vi "Just video.vi"() -> ()   [LabVIEW 2014]
uses:
  <vilib>/Platform/TimedLoop/XDataNode/wakeup.ctl
  <vilib>/Platform/TimedLoop/XDataNode/XDNodeRunTimeDep.lvlib
  <vilib>/Platform/TimedLoop/XDataNode/nitl_modes.ctl
  <vilib>/Platform/TimedLoop/XDataNode/timing_clust.ctl
  <vilib>/Platform/TimedLoop/XDataNode/XDataNode.xnode
  <vilib>/vision/Avi1.llb/AviRefnum.ctl
panel:
  out "Image 2":T1(plugin-control)
  in  "Image Index":dbl=1.0 min=1.0
  in  "Capture and Save Image":bool
  in  "Averaging":bool
  in  "Reset Averaging":bool
  in  "Capture Video":bool
  out "Image":u32[][](graph)
  in  "Intensity Upper":u8=88
  in  "Intensity Lower":u8=66
  in  "Initial Window Size":cluster{"Width":i32, "Height":i32}={"Width"=884, "Height"=619}
  in  "Initial Window Position":cluster{"X Position":i32, "Y Position":i32}={"X Position"=796, "Y Position"=4}
  in  "Zoom Factor":sgl=7.0
  in  "Center Point":cluster{"X":i32, "Y":i32}={"X"=335, "Y"=271}
  out "Window Size":cluster{"Width":i32, "Height":i32}
  out "Window Position":cluster{"X Position":i32, "Y Position":i32}={"X Position"=40, "Y Position"=40}
  in  "New Video File":bool
  in  "Video Index":dbl=1.0 min=1.0 step=1.0
  out "Path Out":path
  in  "Video Capture Rate (Hz)":dbl=30.0
  in  "Stop All":bool
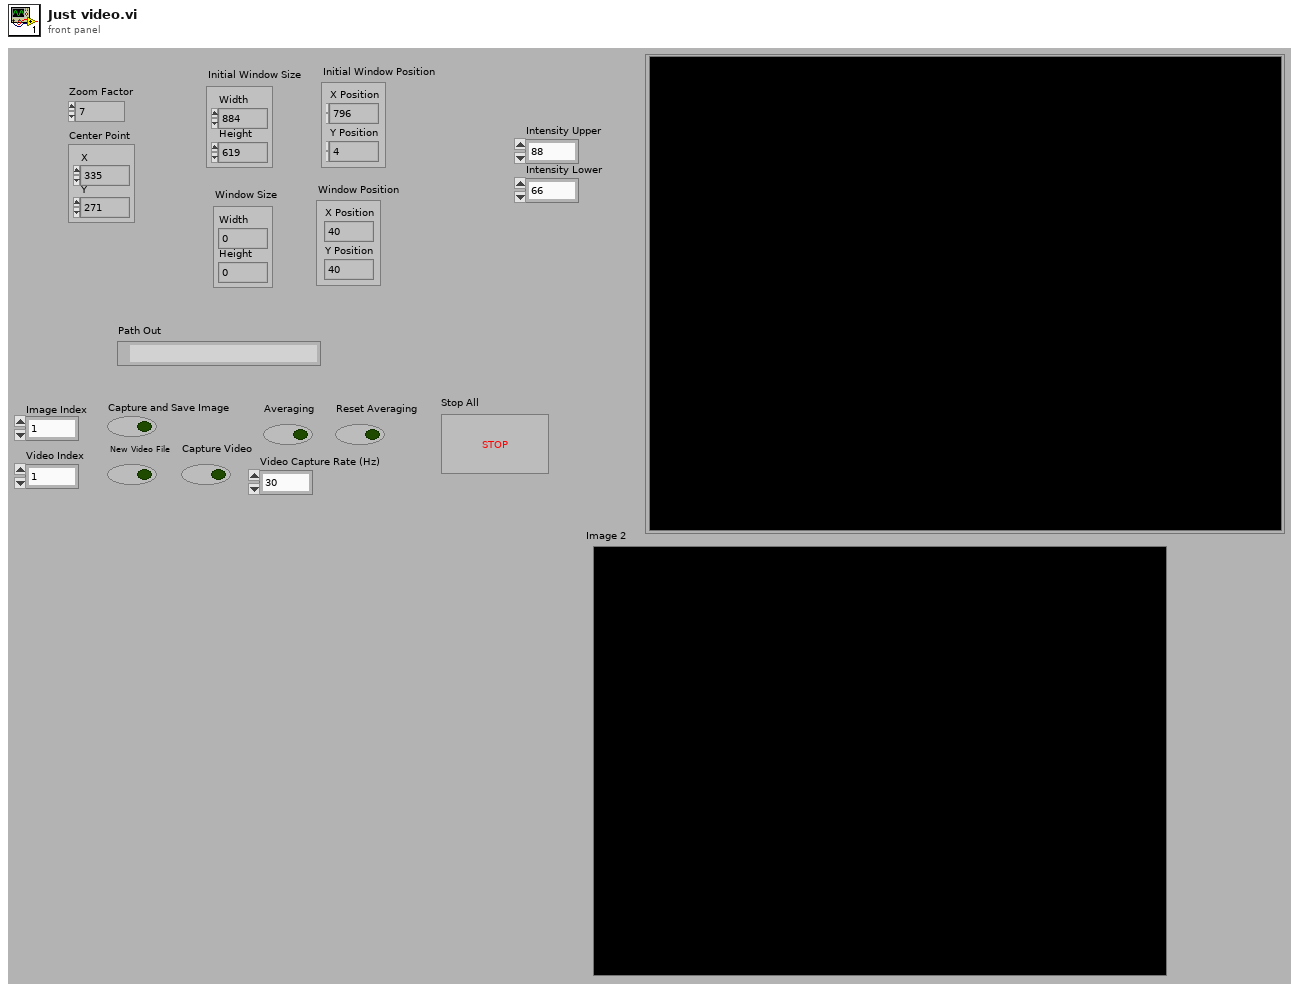
[diagram p1: front panel]
types:
  T1 = typedef "IMAQ Image.ctl" = refnum<image>
  T2 = enum32{"setting", "request", "request control", "info", "statistics", "system settings", "I/O sub system", "HRT control", "camera descriptions", "device specific data", "event sub system settings", "event sub system results", "image memory manager"}
  T3 = typedef "AviRefnum.ctl" = refnum<k1>
  T4 = typedef "XDNodeRunTimeDep.lvlib/timing_clust.ctl" = cluster{"Expected End [f-1]":u64, "Actual End [f-1]":u64, "Finished Late? [f-1]":bool, "Expected End [i-1]":u64, "Actual End [i-1]":u64, "Finished Late? [i-1]":bool, "Expected Start [i]":u64, "Actual Start [i]":u64, "Expected Start [f]":u64, "Actual Start [f]":u64, "Source Name":string, "Structure Name":string, "Period":i64, "Deadline":i64, "Offset":i64, "Start":i64, "Priority":i32, "Timeout":i32, "Mode":T5, "Wakeup Reason":T6, "Error":errorcluster, "Source Type":string, "Secondary Source Type":string, "Global End Time":u64, "Global Start Time":u64, "Frame Duration":u64, "Iteration Duration":u64, "Assigned CPU":i32, "I/O Scan Engine Mode":u32}
  T5 = typedef "XDNodeRunTimeDep.lvlib/nitl_modes.ctl" = enum32{"No Change", "Process missed periods, maintain original phase", "Discard missed periods, maintain original phase", "Process missed periods, ignore original phase", "Discard missed periods, ignore original phase"}
  T6 = typedef "XDNodeRunTimeDep.lvlib/wakeup.ctl" = enum32{"Normal", "Aborted", "Asynchronous wakeup", "Timing source error", "Timed loop error", "Timeout"}
  T7 = typedef "Image Type" = u32
  T8 = typedef "imagedata.ctl" = cluster{"image type":i32, "image depth":i32, "image":u8[], "mask":u8[], "colors":u32[], "Rectangle":cluster{"left":i16, "top":i16, "right":i16, "bottom":i16}}
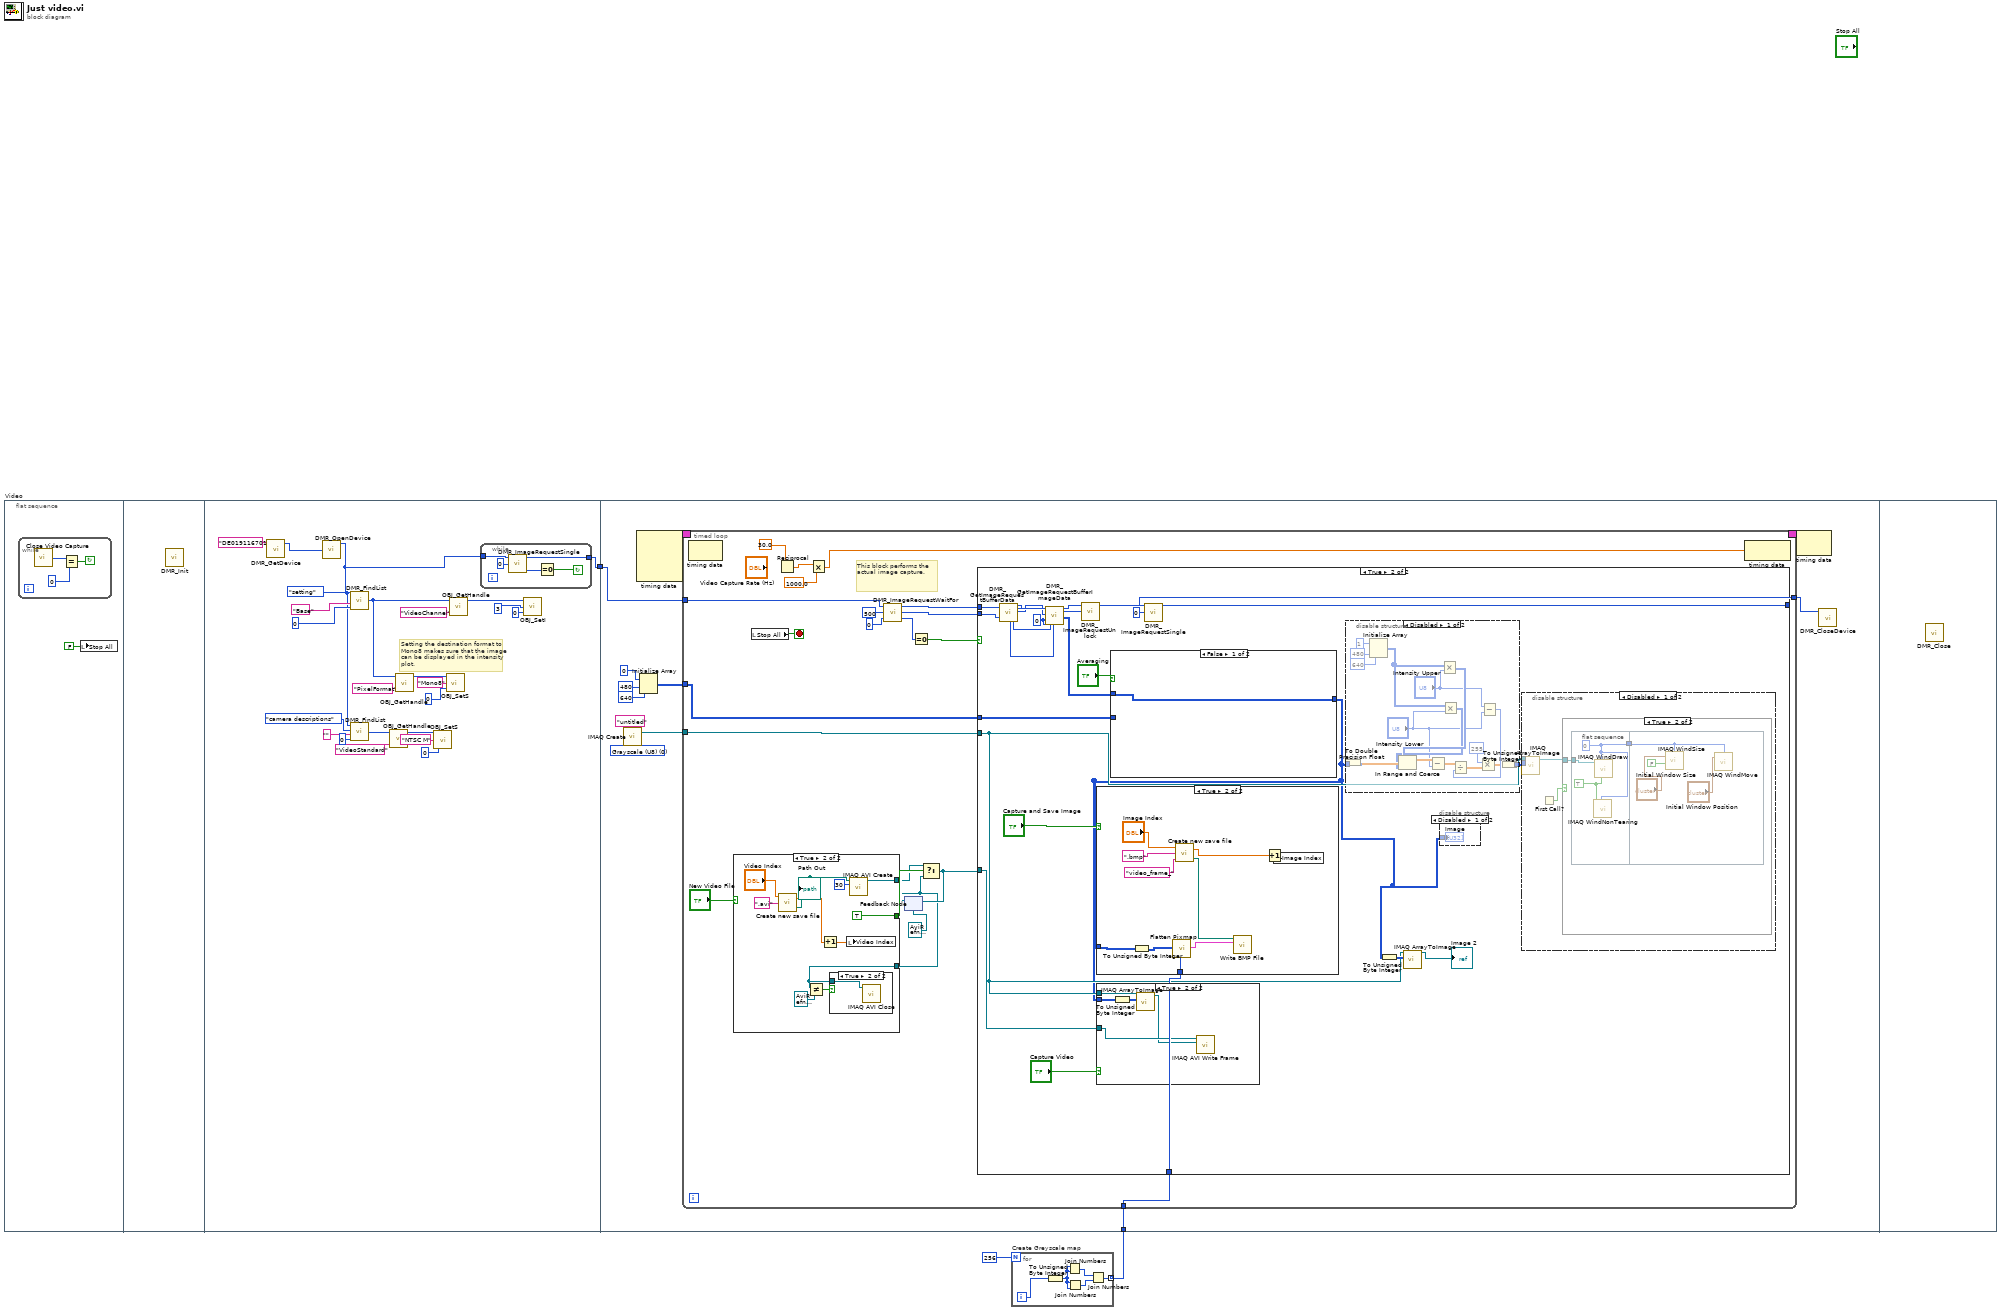
[diagram p0: block diagram]
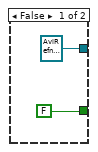
[diagram p2: hidden frame]
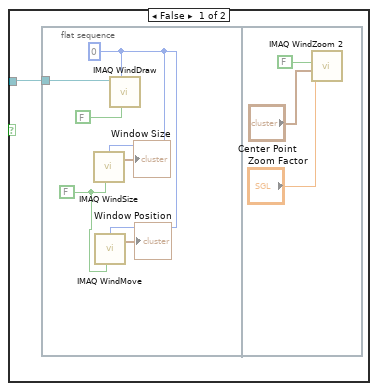
[diagram p7: hidden frame]
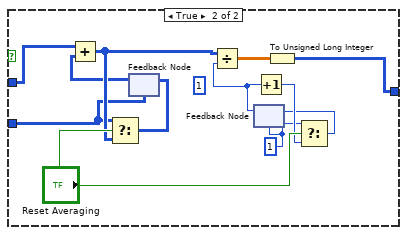
[diagram p10: hidden frame]
diagram:
  n1 = flat-sequence "Video" {
    tunnel: [w12] -> w3
    tunnel: w3 -> [w48]
    tunnel: w1 -> [w46]
    frame #0 {
      n2 = while {
        stop <- w5 continue-if-true
        n3 = call "Close Video Capture.vi"() -> ("error code OUT"=w7:i32)
        n4 = Equal?(x=w7, y=0) -> (x = y?=w5:bool)
      }
      n5 = local write "Stop All"(FALSE ("Stop All")) -> ()
    }
    frame #1 {
      n6 = call "DMR_Init.vi"() -> ()  [unwired: 3 out]
    }
    frame #2 {
      # "Setting the destination format to Mono8 makes sure that the image can be displayed in the intensity plot."
      n7 = call "DMR_GetDevice.vi"("search string IN"="DE019116701") -> ("device handle OUT"=w30:i32)  [unwired: 4 in, 2 out]
      n8 = call "DMR_OpenDevice.vi"("device handle IN"=w30) -> ("driver handle OUT"=w13:i32)  [unwired: 4 out]
      n9 = call "DMR_FindList.vi"("flags IN"=u32 0 ("flags"), "list name IN"="" ("String"), "list type IN"=T2."camera descriptions", "driver handle IN"=w13) -> ("list handle OUT"=w16:i32)  [unwired: 2 out]
      n10 = call "DMR_FindList.vi"("flags IN"=u32 0 ("flags"), "list name IN"="Base", "list type IN"=T2."setting", "driver handle IN"=w13) -> ("list handle OUT"=w14:i32)  [unwired: 2 out]
      n11 = call "OBJ_GetHandle.vi"("object name IN"="VideoStandard", "list handle IN"=w16) -> ("object handle OUT"=w10:i32)  [unwired: 3 out]
      n12 = call "OBJ_GetHandle.vi"("object name IN"="PixelFormat", "list handle IN"=w14) -> ("object handle OUT"=w24:i32)  [unwired: 3 out]
      n13 = call "OBJ_SetS.vi"("value index IN"=0, "value IN"="NTSC M", "object handle IN"=w10) -> ()  [unwired: 2 out]
      n14 = call "OBJ_SetS.vi"("value index IN"=0, "value IN"="Mono8" ("value"), "object handle IN"=w24) -> ()  [unwired: 2 out]
      n15 = call "OBJ_GetHandle.vi"("object name IN"="VideoChannel", "list handle IN"=w14) -> ("object handle OUT"=w20:i32)  [unwired: 3 out]
      n16 = while {
        tunnel: [w35] -> w12
        tunnel: w13 -> [w32]
        stop <- w33 continue-if-true
        n17 = call "DMR_ImageRequestSingle.vi"("request control IN"=0, "driver handle IN"=w32) -> ("error code OUT"=w34:i32, "driver handle OUT"=w35:i32)  [unwired: 2 out]
        n18 = Equal To 0?(x=w34) -> (x = 0?=w33:bool)
      }
      n19 = call "OBJ_SetI.vi"("value index IN"=0, "value IN"=3 ("Video channel"), "object handle IN"=w20) -> ()  [unwired: 2 out]
    }
    frame #3 {
      w43 = T7 0 items=["Grayscale (U8)", "Grayscale (I16)", "Grayscale (SGL)", "Complex (CSG)", "RGB (U32)", "HSL (U32)", "RGB (U64)"] ("Image Type")
      n20 = call "IMAQ Create"("Image Name"="untitled", "Image Type"=w43) -> ("New Image"=w44:T1)  [unwired: 2 in, 2 out]
      n21 = node-c288() -> (w42:T4)  [unwired: 4 out]
      n22 = Initialize Array(u32 0 ("Window Number (0...15)"), 480 ("dimension size"), 640 ("dimension size")) -> (w37:u32[][])
      n23 = timed-loop {
        tunnel: w48 -> [w64]
        tunnel: [w63] -> w47
        tunnel: w46 -> [w62]
        tunnel: w44 -> [w61]
        timing: w42 -> [_]
        timing-out: [_] -> w41
        tunnel: w37 -> [w51]
        stop <- w49 stop-if-true
        # "This block performs the \nactual image capture."
        n24 = node-c288() -> ()  [unwired: 2 out]
        n25 = local read "Stop All"() -> (w49:bool)
        n26 = Reciprocal(x=30.0) -> (1/x=w54:dbl)
        n27 = Multiply(x=w54, y=1000.0) -> (x*y=w52:dbl)
        n28 = call "DMR_ImageRequestWaitFor.vi"("queue number IN"=0, "timeout(ms) IN"=500, "driver handle IN"=w64) -> ("error code OUT"=w68:i32, "request number OUT"=w65:i32, "driver handle OUT"=w66:i32)
        n29 = feedback #1(T3 refnum ("Avi Refnum")) -> (w55:T3)
        n30 = case shown="True" "New Video File" {
          tunnel: [T3 refnum ("Avi Refnum") w85] -> w57
          tunnel: [FALSE TRUE] -> w58
          tunnel: w55 -> [_ w81]
          frame False {
          }
          frame True {
            n31 = call "Create new save file.vi"("Ext"=".avi" ("string"), "Index In"="Video Index") -> ("Path Out"=w77:path, "Index Out"=w78:dbl)  [unwired: 1 in]
            "Path Out" <- w77
            n32 = Not Equal?(x=w81, y=T3 refnum ("Avi Refnum")) -> (x != y?=w82:bool)
            n33 = Increment(x=w78) -> (x+1=w87:dbl)
            n34 = case shown="True" w82 {
              tunnel: w81 -> [_ w88]
              frame False {
              }
              frame True {
                n35 = call "IMAQ AVI Close"("Avi Refnum"=w88) -> ()  [unwired: 1 in, 10 out]
              }
            }
            n36 = local write "Video Index"(w87) -> ()
            n37 = call "IMAQ AVI Create"("Frames Per Second"=u32 30, "AVI Path"=w77) -> ("Avi Refnum"=w85:T3)  [unwired: 5 in, 4 out]
          }
        }
        n38 = Equal To 0?(x=w68) -> (x = 0?=w67:bool)
        n39 = Select(t=w57, s=w58, f=w55) -> (s? t:f=w56:T3)
        n40 = feedback-in #1(w56) -> ()
        n41 = case shown="True" w67 {
          tunnel: w66 -> [w89 w114]
          tunnel: w65 -> [_ w113]
          tunnel: [w89 w110] -> w63
          tunnel: w62 -> [_ w100]
          tunnel: w61 -> [_ w92]
          tunnel: w51 -> [_ w97]
          tunnel: w56 -> [_ w95]
          frame False {
          }
          frame True {
            w104 = u32 0 ("X-offset IN")
            n42 = call "DMR_GetImageRequestBufferData.vi"("driver handle IN"=w114, "request number IN"=w113) -> ("width OUT"=w103:i32, "height OUT"=w102:i32, "driver handle OUT"=w109:i32, "request number OUT"=w108:i32, "bytes per pixel OUT"=w105:i32)  [unwired: 13 out]
            n43 = call "DMR_GetImageRequestBufferImageData.vi"("driver handle IN"=w109, "request number IN"=w108, "bytes per pixel IN"=w105, "X-offset IN"=w104, "Y-offset IN"=w104, "height IN"=w102, "width IN"=w103) -> ("driver handle OUT"=w107:u32, "request number OUT"=w106:u32, "image OUT"=w98:u32[][])  [unwired: 10 out]
            n44 = call "DMR_ImageRequestUnlock.vi"("request number IN"=w106, "driver handle IN"=w107) -> ("driver handle OUT"=w112:i32)  [unwired: 1 in, 2 out]
            n45 = case shown="False" "Averaging" {
              tunnel: w98 -> [w161 w166]
              tunnel: [w161 w165] -> w90
              tunnel: w97 -> [_ w163]
              frame False {
              }
              frame True {
                (unwired) 1
                w171 = 1
                n46 = feedback #2(w163) -> (w162:u32[][])
                n47 = Add(x=w166, y=w162) -> (x+y=w167:u32[][])
                n48 = Select(t=w163, s="Reset Averaging", f=w167) -> (s? t:f=w169:u32[][])
                n49 = feedback-in #2(w169) -> ()
                n50 = feedback #3(w171) -> (w164:i32)
                n51 = Divide(x=w167, y=w164) -> (x/y=w168:dbl[][])
                n52 = Increment(x=w164) -> (x+1=w172:i32)
                n53 = To Unsigned Long Integer(number=w168) -> (unsigned 32bit integer=w165:u32[][])
                n54 = Select(t=w171, s="Reset Averaging", f=w172) -> (s? t:f=w170:i32)
                n55 = feedback-in #3(w170) -> ()
              }
            }
            n56 = case shown="True" "Capture and Save Image" {
              tunnel: w90 -> [_ w183]
              tunnel: w100 -> [_ w182]
              frame False {
              }
              frame True {
                n57 = To Unsigned Byte Integer(number=w183) -> (unsigned 8bit integer=w179:u8[][])
                n58 = call <vilib>:"Flatten Pixmap.vi"("colors"=w182, "8-bit pixmap"=w179) -> ("image data"=w180:T8)  [unwired: 4 in, 5 out]
                n59 = call "Create new save file.vi"("Insert"="video_frame_" ("string"), "Ext"=".bmp" ("string"), "Index In"="Image Index") -> ("Path Out"=w175:path, "Index Out"=w181:dbl)
                n60 = call <vilib>:"Write BMP File.vi"("image data"=w180, "path to BMP file"=w175) -> ()  [unwired: 1 in, 9 out]
                n61 = Increment(x=w181) -> (x+1=w174:dbl)
                n62 = local write "Image Index"(w174) -> ()
              }
            }
            n63 = case shown="True" "Capture Video" {
              tunnel: w95 -> [_ w160]
              tunnel: w90 -> [_ w158]
              tunnel: w92 -> [_ w157]
              frame False {
              }
              frame True {
                n64 = To Unsigned Byte Integer(number=w158) -> (unsigned 8bit integer=w159:u8[][])
                n65 = call "IMAQ ArrayToImage"("Image Pixels (U8)"=w159, "Image"=w157) -> ("Image Out"=w156:T1)  [unwired: 4 in, 5 out]
                n66 = call "IMAQ AVI Write Frame"("Image"=w156, "Avi Refnum"=w160) -> ()  [unwired: 2 in, 8 out]
              }
            }
            n67 = call "DMR_ImageRequestSingle.vi"("request control IN"=0, "driver handle IN"=w112) -> ("driver handle OUT"=w110:i32)  [unwired: 3 out]
            n68 = disable-structure shown="Disabled" {
              disable-tunnel: w90 -> [w132 _]
              disable-tunnel: [w116 _] -> w94
              frame Disabled {
                n69 = To Double Precision Float(number=w132) -> (double precision float=w128:dbl[][])
                n70 = Initialize Array(u8 1, 480 ("dimension size"), 640 ("dimension size")) -> (w127:u8[][])
                n71 = Multiply(x=w127, y="Intensity Upper") -> (x*y=w126:u8[][])
                n72 = Multiply(x=w127, y="Intensity Lower") -> (x*y=w125:u8[][])
                n73 = In Range and Coerce(upper limit=w126, x=w128, lower limit=w125) -> (coerced(x)=w124:dbl[][])  [unwired: 1 out]
                n74 = Subtract(x=w124, y="Intensity Lower") -> (x-y=w120:dbl[][])
                n75 = Subtract(x="Intensity Upper", y="Intensity Lower") -> (x-y=w119:u8)
                n76 = Divide(x=w120, y=w119) -> (x/y=w121:dbl[][])
                n77 = Multiply(x=u8 255, y=w121) -> (x*y=w117:dbl[][])
                n78 = To Unsigned Byte Integer(number=w117) -> (unsigned 8bit integer=w116:u8[][])
              }
              frame Enabled {
              }
            }
            n79 = To Unsigned Byte Integer(number=w90) -> (unsigned 8bit integer=w93:u8[][])
            n80 = call "IMAQ ArrayToImage"("Image Pixels (U8)"=w93, "Image"=w92) -> ("Image Out"=→"Image 2":T1)  [unwired: 4 in, 5 out]
            n81 = disable-structure shown="Disabled" {
              disable-tunnel: w90 -> [w115 _]
              frame Disabled {
                "Image" <- w115
              }
              frame Enabled {
              }
            }
            n82 = disable-structure shown="Disabled" {
              disable-tunnel: w92 -> [w136 _]
              disable-tunnel: w94 -> [w133 _]
              frame Disabled {
                n83 = call "IMAQ ArrayToImage"("Image Pixels (U8)"=w133, "Image"=w136) -> ("Image Out"=w134:T1)  [unwired: 4 in, 5 out]
                n84 = First Call?() -> (First Call?: T/F=w135:bool)
                n85 = case shown="True" w135 {
                  tunnel: w134 -> [w137 w148]
                  frame False {
                    n86 = flat-sequence {
                      tunnel: w137 -> [w143]
                      frame #0 {
                        w140 = FALSE ("Get/Set Status? (Set)")
                        w139 = 0 ("Window Number (0...15)")
                        n87 = call "IMAQ WindSize"("Get/Set Status? (Set)"=w140, "Window Number"=w139) -> ("Width & Height out"=→"Window Size":cluster{"Width":i32, "Height":i32})  [unwired: 4 in, 2 out]
                        n88 = call "IMAQ WindMove"("Window Number (0...15)"=w139, "Get/Set Status? (Set)"=w140) -> ("Coordinates (screen)"=→"Window Position":cluster{"X Position":i32, "Y Position":i32})  [unwired: 3 in, 1 out]
                        n89 = call "IMAQ WindDraw"("Resize to Image Size? (Y)"=FALSE, "Window Number (0...15)"=w139, "Image"=w143) -> ()  [unwired: 7 in, 2 out]
                      }
                      frame #1 {
                        n90 = call "IMAQ WindZoom 2"("Center Point"="Center Point", "Zoom to Fit? (False)"=FALSE, "Zoom Factor"="Zoom Factor") -> ()  [unwired: 5 in, 4 out]
                      }
                    }
                  }
                  frame True {
                    n91 = flat-sequence {
                      tunnel: w148 -> [w151]
                      tunnel: [w149] -> w147
                      tunnel: w147 -> [w153]
                      frame #0 {
                        w150 = TRUE ("Resize to Image Size? (Y)")
                        w149 = 0 ("Window Number (0...15)")
                        n92 = call "IMAQ WindNonTearing"("Window Number"=w149, "NonTearing? (True)"=w150) -> ()  [unwired: 8 in, 2 out]
                        n93 = call "IMAQ WindDraw"("Resize to Image Size? (Y)"=w150, "Window Number (0...15)"=w149, "Image"=w151) -> ()  [unwired: 7 in, 2 out]
                      }
                      frame #1 {
                        n94 = call "IMAQ WindSize"("Scrollbars? (N)"=FALSE, "Width & Height"="Initial Window Size", "Window Number"=w153) -> ()  [unwired: 3 in, 3 out]
                        n95 = call "IMAQ WindMove"("Window Number (0...15)"=w153, "Coordinates (screen)"="Initial Window Position") -> ()  [unwired: 3 in, 2 out]
                      }
                    }
                  }
                }
              }
              frame Enabled {
              }
            }
          }
        }
        n96 = node-c288(w52) -> ()  [unwired: 1 out]
      }
      n97 = node-c288(w41) -> ()  [unwired: 1 out]
      n98 = call "DMR_CloseDevice.vi"("driver handle IN"=w47) -> ()  [unwired: 1 in, 4 out]
    }
    frame #4 {
      n99 = call "DMR_Close.vi"() -> ()  [unwired: 1 out]
    }
  }
  n100 = for "Create Greyscale map" {
    N: 256 -> [_]
    tunnel: [w187] -> w1 mode=indexing
    i -> [w190]
    n101 = To Unsigned Byte Integer(number=w190) -> (unsigned 8bit integer=w186:u8)
    n102 = Join Numbers(hi=w186, lo=w186) -> ((hi.lo)=w189:u16)
    n103 = Join Numbers(hi=w186, lo=w186) -> ((hi.lo)=w188:u16)
    n104 = Join Numbers(hi=w189, lo=w188) -> ((hi.lo)=w187:u32)
  }
